vi "Autoscan_SavingImagesAndReports.vi"(0 "IntensityGraph in":refnum<vi>, 1 "Measurement Save Path":refnum<vi>, 2 "Array":dbl[][](array[numeric]), 3 "Intensity Graph":dbl[][](array[numeric]), 5 "Color":u32, 7 "Area #":refnum<vi>, 9 "Numeric":i32, 11 "error in (no error)":errorcluster, 12 "quality (80)":i32, 13 "Map centers short":dbl[](array[numeric])) -> (15 "error out":errorcluster)   [LabVIEW 2023]
uses:
  <vilib>/Utility/file.llb/Write Delimited Spreadsheet (DBL).vi
  <vilib>/Utility/file.llb/Write Delimited Spreadsheet (I64).vi
  <vilib>/regexp/Match Regular Expression.xnode
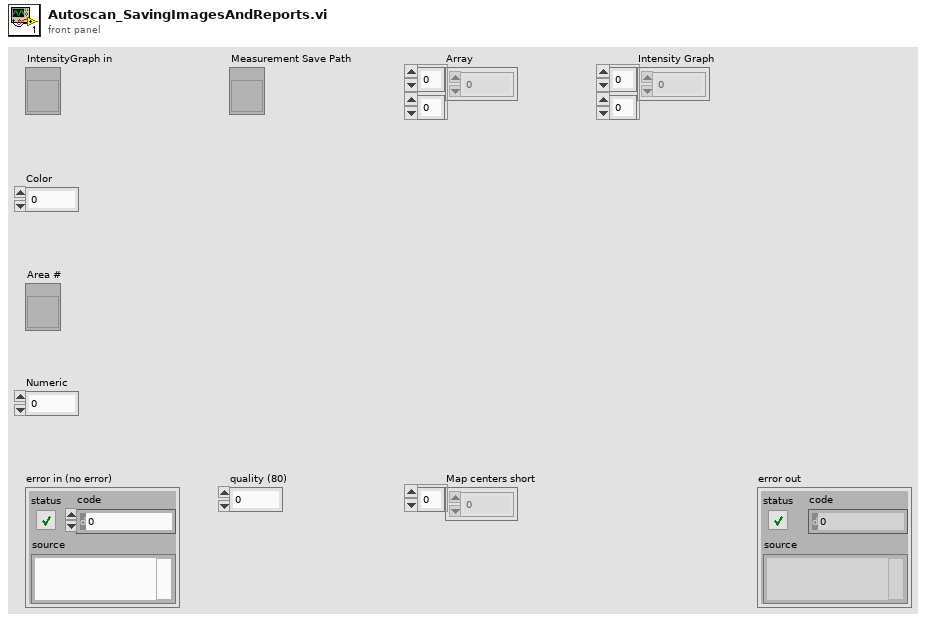
[diagram p1: front panel]
types:
  T1 = typedef "imagedata.ctl" = cluster{"image type":i32, "image depth":i32, "image":u8[], "mask":u8[], "colors":u32[], "Rectangle":cluster{"left":i16, "top":i16, "right":i16, "bottom":i16}}
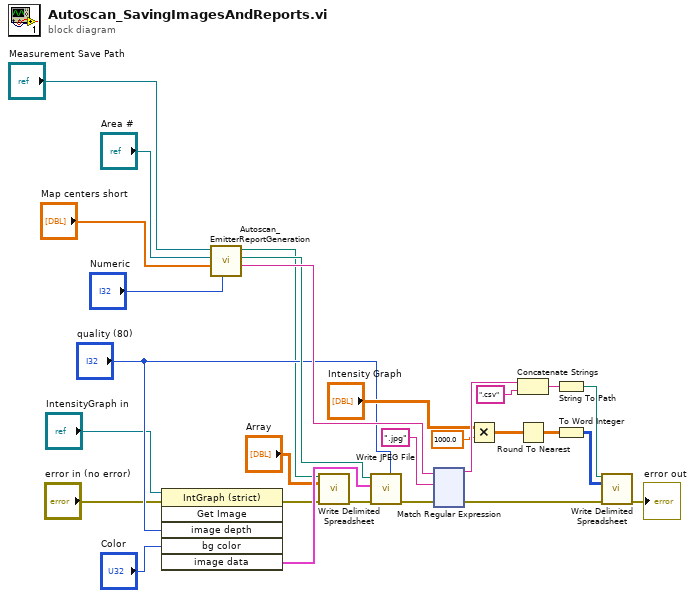
[diagram p0: block diagram]
diagram:
  n1 = invoke on="Invoke Node" class="IntGraph (strict)" method="Get Image"(reference="IntensityGraph in", error in="error in (no error)", "image depth"="quality (80)", "bg color"="Color") -> (error out=w7:errorcluster, "image data"=w8:T1)  [unwired: 2 in, 4 out]
  n2 = call "Autoscan_EmitterReportGeneration.vi"("Numeric"="Numeric", "Map centers short"="Map centers short", "reference in"="Area #", "Path in"="Measurement Save Path") -> ("String"=w20:string, "appended path"=w19:path, "appended path 2"=w2:path)  [unwired: 5 in]
  n3 = call-poly <vilib>:"Write Delimited Spreadsheet.vi"("file path (dialog if empty)"=w2, "2D data"="Array", "error in (no error)"=w7) -> ("error out"=w16:errorcluster)  [unwired: 11 in, 1 out]
  n4 = call <vilib>:"Write JPEG File.vi"("quality (80)"="quality (80)", "error in (no error)"=w16, "image data"=w8, "path to JPEG file"=w19) -> ("error out"=w22:errorcluster)  [unwired: 6 in, 1 out]
  n5 = xnode "Match Regular Expression"("input string"=w20, "regular expression"=".jpg", "error in"=w22) -> ("before match"=w24:string, "error out"=w23:errorcluster)  [unwired: 3 in, 3 out]
  n6 = Multiply(x="Intensity Graph", y=1000.0) -> (x*y=w13:dbl[][])
  n7 = Concatenate Strings(w24, ".csv" ("string")) -> (w26:string)
  n8 = Round To Nearest(number=w13) -> (nearest integer value=w12:dbl[][])
  n9 = String To Path(string=w26) -> (path=w21:path)
  n10 = To Word Integer(number=w12) -> (16bit integer=w11:i16[][])
  n11 = call-poly <vilib>:"Write Delimited Spreadsheet.vi"("file path (dialog if empty)"=w21, "2D data"=w11, "error in (no error)"=w23) -> ("error out"=→"error out":errorcluster)  [unwired: 11 in, 1 out]
